vi "Define Columns.vi"(10 "Enum Array":refnum<vi>[](array[refnum])) -> (2 "Column Definition":T1[](array[typedef]) {"MinWidth" min=2 step=1; "AutoSizeMode" items=["None"=1, "ColumnHeader"=2, "AllCellsExceptHeader"=4, "AllCells"=6, "DisplayedCellsExceptHeader"=8, "DisplayedCells"=10, "Fill"=16]; "FillWeight" min=1 max=100})   [LabVIEW 2015, in "PID Module editor node.lvclass"]
doc: "This VI defines the columns that will be used in the table. You can specify the column type and the dimensions if the columns."
uses:
  PID Module editor node.lvclass
  <vilib>/NI/DCAF/Tag Editor Core/Table API/Column/Column Descriptor.ctl
  <vilib>/NI/DCAF/Tag Editor Core/Table API/Column/Column.lvclass
  <vilib>/NI/DCAF/Tag Editor Core/Table API/Column/Column Type.ctl
  <vilib>/NI/Tag Bus/tag/Data Type.ctl
  <vilib>/NI/DCAF/Tag Editor Core/Table API/Table Manager/Call Back Ref Type Def.ctl
  <vilib>/NI/DCAF/Tag Editor Core/Configuration Editor/Classes/Engine Parent/Engine Parent Editor Node.lvclass
  <vilib>/NI/DCAF/Tag Editor Core/Configuration Editor/Classes/Module editor node/module editor node.lvclass
  module/configuration/String Parameters.ctl
  <vilib>/NI/Tag Bus/tag/tag descriptor.lvclass
  <vilib>/NI/DCAF/Tag Editor Core/Table API/Mapping Column/Mapping Column.lvclass
  <vilib>/NI/DCAF/Tag Editor Core/Table API/String Column/String Column.lvclass
  module/configuration/PID Module configuration.lvclass
  <vilib>/NI/DCAF/Tag Editor Core/Table API/Table Manager/Table Manager.lvclass
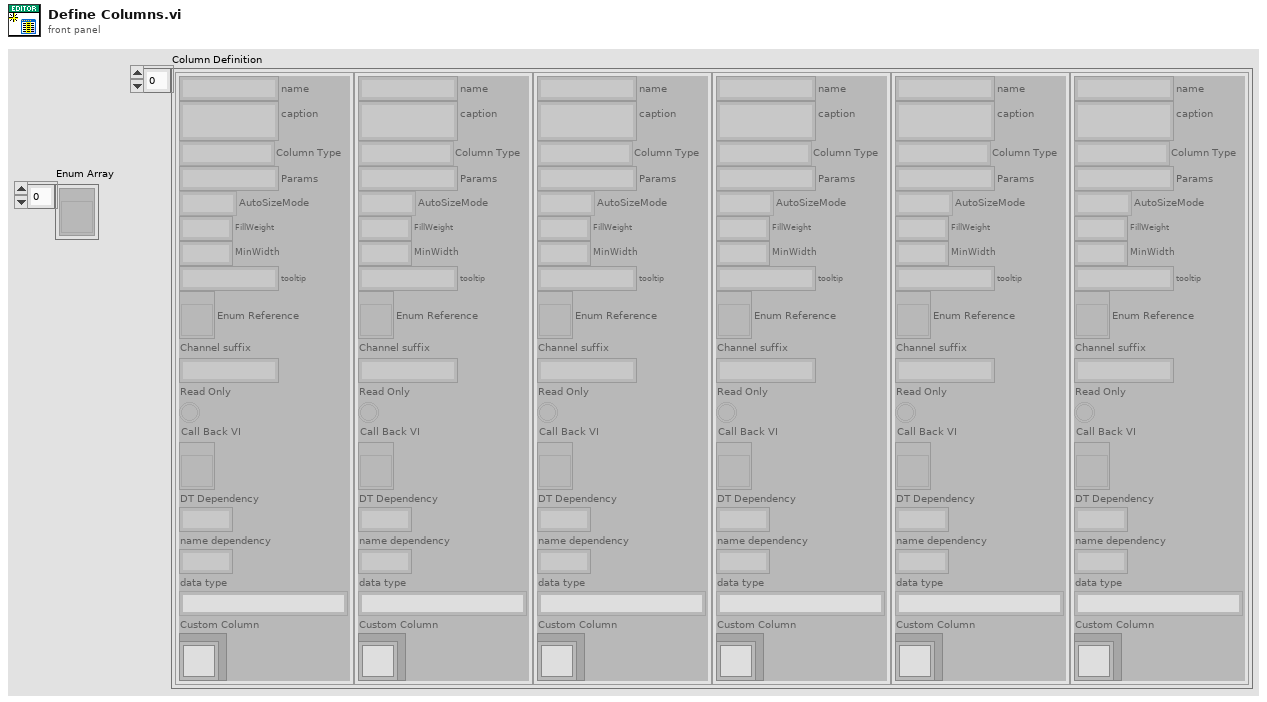
[diagram p1: front panel]
types:
  T1 = typedef "Table Manager.lvlib/Column.lvclass/Column Descriptor.ctl" = cluster{"name":string, "caption":string, "Column Type":T2, "Params":string, "AutoSizeMode":i32, "FillWeight":sgl, "MinWidth":u32, "tooltip":string, "Enum Reference":refnum<vi>, "Channel suffix":string, "Read Only":bool, "Call Back VI":T3, "DT Dependency":i32, "name dependency":i32, "data type":T4, "Custom Column":refnum<class "Column.lvclass">}
  T2 = typedef "Table Manager.lvlib/Column.lvclass/Column Type.ctl" = enum16{"String", "Mapping", "Enum", "Custom"}
  T3 = typedef "Table Manager.lvlib/Table Manager.lvclass/Call Back Ref Type Def.ctl" = refnum<vi>
  T4 = typedef "tag bus.lvlib/tag descriptor.lvclass/Data Type.ctl" = enum16{"Double", "Single", "I64", "I32", "I16", "I8", "U64", "U32", "U16", "U8", "Boolean", "String", "Array of Double", "Array of Single", "Array of I64", "Array of I32", "Array of I16", "Array of I8", "Array of U64", "Array of U32", "Array of U16", "Array of U8", "Array of Boolean", "Array of String"}
  T5 = typedef "PID Module configuration.lvclass/String Parameters.ctl" = enum16{"Setpoint", "Process Variable", "Output", "Proportional Gain", "Integral Time", "Derivative Time", "Range High", "Range Low"}
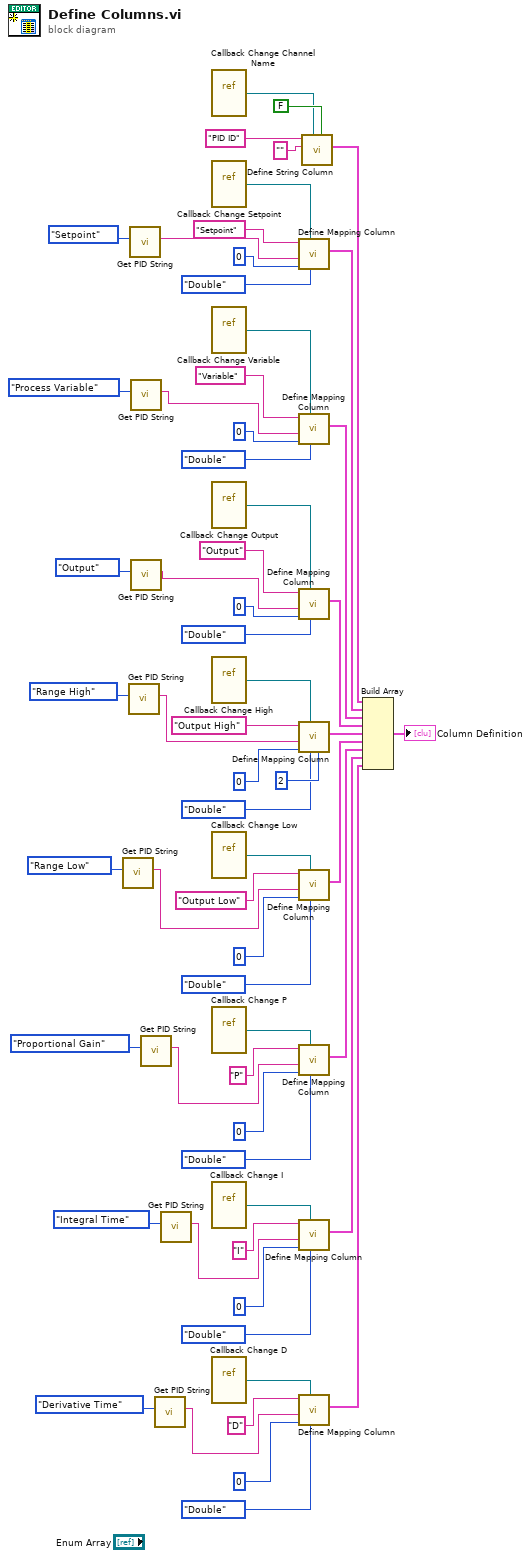
[diagram p0: block diagram]
diagram:
  n1 = call "Get PID String.vi"("PID Parameter"=String_Parameters."Range Low") -> ("Parameter String"=w3:string)  [unwired: 8 in]
  n2 = call "Get PID String.vi"("PID Parameter"=String_Parameters."Range High") -> ("Parameter String"=w4:string)  [unwired: 8 in]
  n3 = call "Get PID String.vi"("PID Parameter"=String_Parameters."Setpoint") -> ("Parameter String"=w15:string)  [unwired: 8 in]
  n4 = call "Get PID String.vi"("PID Parameter"=String_Parameters."Process Variable") -> ("Parameter String"=w6:string)  [unwired: 8 in]
  n5 = call "Get PID String.vi"("PID Parameter"=String_Parameters."Output") -> ("Parameter String"=w5:string)  [unwired: 8 in]
  n6 = call "Get PID String.vi"("PID Parameter"=String_Parameters."Proportional Gain") -> ("Parameter String"=w2:string)  [unwired: 8 in]
  n7 = call "Get PID String.vi"("PID Parameter"=String_Parameters."Derivative Time") -> ("Parameter String"=w7:string)  [unwired: 8 in]
  n8 = call "Get PID String.vi"("PID Parameter"=String_Parameters."Integral Time") -> ("Parameter String"=w1:string)  [unwired: 8 in]
  n9 = vi-ref "Callback Change Channel Name.vi"() -> (w54:refnum<vi>)
  n10 = vi-ref "Callback Change Setpoint.vi"() -> (w49:refnum<vi>)
  n11 = vi-ref "Callback Change Variable.vi"() -> (w48:refnum<vi>)
  n12 = vi-ref "Callback Change Output.vi"() -> (w63:refnum<vi>)
  n13 = vi-ref "Callback Change High.vi"() -> (w40:refnum<vi>)
  n14 = vi-ref "Callback Change Low.vi"() -> (w26:refnum<vi>)
  n15 = vi-ref "Callback Change P.vi"() -> (w25:refnum<vi>)
  n16 = vi-ref "Callback Change I.vi"() -> (w24:refnum<vi>)
  n17 = vi-ref "Callback Change D.vi"() -> (w21:refnum<vi>)
  n18 = call <vilib>:"Define Mapping Column.vi"("data type"=Data_Type."Double", "Call Back VI"=w49, "name dependency"=0, "Channel suffix"=w15, "name"="Setpoint") -> ("Column Descriptor out"=w39:T1)  [unwired: 6 in]
  n19 = call <vilib>:"Define Mapping Column.vi"("data type"=Data_Type."Double", "Call Back VI"=w48, "name dependency"=0, "Channel suffix"=w6, "name"="Variable") -> ("Column Descriptor out"=w38:T1)  [unwired: 6 in]
  n20 = call <vilib>:"Define Mapping Column.vi"("data type"=Data_Type."Double", "Call Back VI"=w63, "name dependency"=0, "Channel suffix"=w5, "name"="Output") -> ("Column Descriptor out"=w53:T1)  [unwired: 6 in]
  n21 = call <vilib>:"Define Mapping Column.vi"("DT Dependency (-1)"=2 ("DT Dependency"), "data type"=Data_Type."Double", "Call Back VI"=w40, "name dependency"=0, "Channel suffix"=w4, "name"="Output High") -> ("Column Descriptor out"=w37:T1)  [unwired: 5 in]
  n22 = call <vilib>:"Define Mapping Column.vi"("data type"=Data_Type."Double", "Call Back VI"=w26, "name dependency"=0, "Channel suffix"=w3, "name"="Output Low") -> ("Column Descriptor out"=w27:T1)  [unwired: 6 in]
  n23 = call <vilib>:"Define Mapping Column.vi"("data type"=Data_Type."Double", "Call Back VI"=w25, "name dependency"=0, "Channel suffix"=w2, "name"="P") -> ("Column Descriptor out"=w23:T1)  [unwired: 6 in]
  n24 = call <vilib>:"Define Mapping Column.vi"("data type"=Data_Type."Double", "Call Back VI"=w24, "name dependency"=0, "Channel suffix"=w1, "name"="I") -> ("Column Descriptor out"=w22:T1)  [unwired: 6 in]
  n25 = call <vilib>:"Define Mapping Column.vi"("data type"=Data_Type."Double", "Call Back VI"=w21, "name dependency"=0, "Channel suffix"=w7, "name"="D") -> ("Column Descriptor out"=w17:T1)  [unwired: 6 in]
  n26 = call <vilib>:"Define String Column.vi"("Read Only (F)"=FALSE ("Read Only"), "Call Back VI"=w54, "Caption"="", "Name"="PID ID" ("name")) -> ("Column Descriptor out"=w56:T1)  [unwired: 7 in]
  n27 = Build Array(w56, w39, w38, w53, w37, w27, w23, w22, w17) -> (→"Column Definition":T1[])
